vi "Query Chan Parameters (Output).vi"(7 "Channel (1: Chan A)":i32(ring)=1 items=["Channel A"=1, "Channel B"=2, "Channel C"=3, "Channel D"=4, "Channel E"=5, "Channel F"=6, "Channel G"=7, "Channel H"=8], 8 "error in (no error)":errorcluster, 11 "VISA resource name":refnum<visa-resource-name>) -> (0 "error out":errorcluster, 2 "Output Parameters":T1={"Polarity Out"=FALSE, "Level Value"=nan, "Level Out"=enum."TTL", "MUX Value"=0} {"Level Value" format="%.3p"}, 3 "VISA resource name out":refnum<visa-resource-name>)   [LabVIEW 2019, in "Quantum Composers 9000 Series.lvlib"]
doc: "This VI is used to read the output configuration of the selected channel."
uses:
  Quantum Composers 9000 Series.lvlib
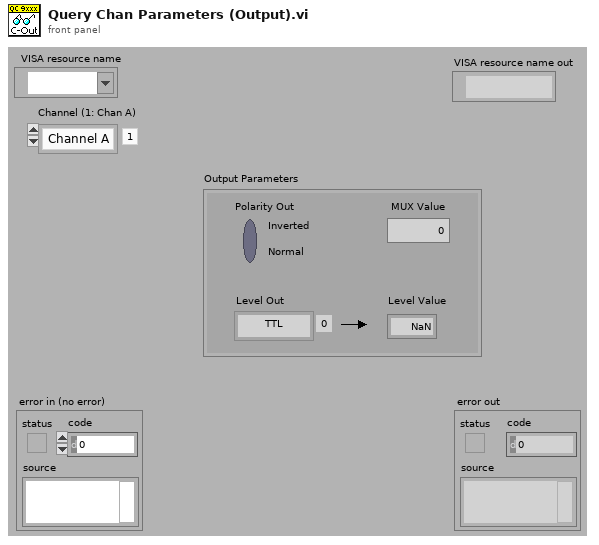
[diagram p1: front panel]
types:
  T1 = cluster{"Polarity Out":bool, "Level Value":dbl, "Level Out":enum16{"TTL", "Adjustable", "35 Volt", "Optical"}, "MUX Value":i32}
  T2 = enum16{"TTL", "Adjustable", "35 Volt", "Optical"}
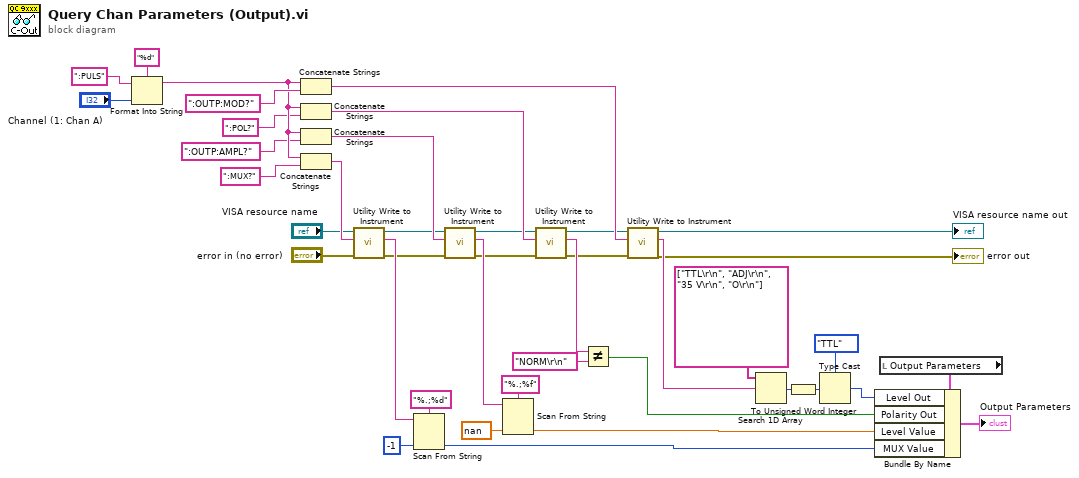
[diagram p0: block diagram]
diagram:
  n1 = Format Into String(format string="%d", initial string=":PULS", "Channel (1: Chan A)") -> (resulting string=w33:string)  [unwired: 1 in, 1 out]
  n2 = Concatenate Strings(w33, ":OUTP:MOD?") -> (w26:string)
  n3 = Concatenate Strings(w33, ":POL?") -> (w27:string)
  n4 = Concatenate Strings(w33, ":OUTP:AMPL?") -> (w28:string)
  n5 = Concatenate Strings(w33, ":MUX?") -> (w29:string)
  n6 = call "Utility Write to Instrument.vi"("error in (no error)"="error in (no error)", "Write Buffer"=w29, "VISA resource name"="VISA resource name") -> ("error out"=w23:errorcluster, "Read Buffer"=w38:string, "VISA resource name out"=w22:refnum<visa-resource-name>)  [unwired: 6 in]
  n7 = Scan From String(format string="%.;%d", input string=w38, default 1=-1 ("default value 1")) -> (output 1=w9:i32)  [unwired: 2 in, 3 out]
  n8 = call "Utility Write to Instrument.vi"("error in (no error)"=w23, "Write Buffer"=w28, "VISA resource name"=w22) -> ("error out"=w14:errorcluster, "Read Buffer"=w21:string, "VISA resource name out"=w13:refnum<visa-resource-name>)  [unwired: 6 in]
  n9 = Scan From String(format string="%.;%f", input string=w21, default 1=nan ("default value 1")) -> (output 1=w7:dbl)  [unwired: 2 in, 3 out]
  n10 = call "Utility Write to Instrument.vi"("error in (no error)"=w14, "Write Buffer"=w27, "VISA resource name"=w13) -> ("error out"=w15:errorcluster, "Read Buffer"=w19:string, "VISA resource name out"=w16:refnum<visa-resource-name>)  [unwired: 6 in]
  n11 = Not Equal?(x=w19, y="NORM\r\n") -> (x != y?=w8:bool)
  n12 = call "Utility Write to Instrument.vi"("error in (no error)"=w15, "Write Buffer"=w26, "VISA resource name"=w16) -> ("error out"=→"error out":errorcluster, "Read Buffer"=w17:string, "VISA resource name out"=→"VISA resource name out":refnum<visa-resource-name>)  [unwired: 6 in]
  n13 = Search 1D Array(1D array=string[] ["TTL\r\n", "ADJ\r\n", "35 V\r\n", "O\r\n"], element=w17) -> (index of element=w1:i32)  [unwired: 1 in]
  n14 = To Unsigned Word Integer(number=w1) -> (unsigned 16bit integer=w2:u16)
  n15 = Type Cast(type=T2."TTL" ("Level Out"), x=w2) -> (*(type *) &x=w3:T2)
  n16 = local read "Output Parameters"() -> (w5:T1)
  n17 = Bundle By Name(cluster=w5, "Level Out"=w3, "Polarity Out"=w8, "Level Value"=w7, "MUX Value"=w9) -> (→"Output Parameters":T1)
